vi "adjust_default_pressure.vi"(11 "Set Pressure Cluster":T1={"Control Pressure"=268.93469325770803, "Set Water Mix Pressures"=[nan, nan, nan, 501.0563822038507, 515.6849104636661, 529.5698810290002, 543.7581328797552, 555.1850771044066, 568.1044613714394], "Set Odor Pressures"=[nan, nan, 465.17755108085316, 474.38001525731295]}) -> (3 "new default pressure":dbl[](array[numeric]))   [LabVIEW 2016]
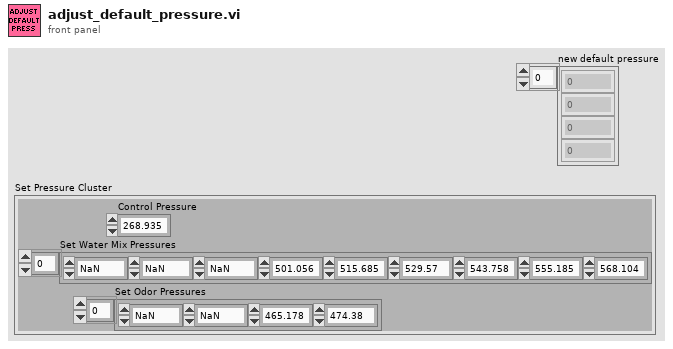
[diagram p1: front panel]
types:
  T1 = cluster{"Control Pressure":dbl, "Set Water Mix Pressures":dbl[], "Set Odor Pressures":dbl[]}
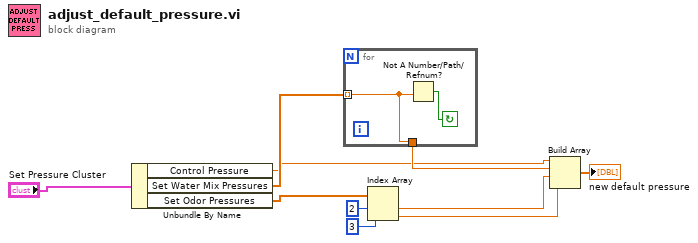
[diagram p0: block diagram]
diagram:
  n1 = Unbundle By Name("Set Pressure Cluster") -> ("Control Pressure"=w2:dbl, "Set Water Mix Pressures"=w4:dbl[], "Set Odor Pressures"=w9:dbl[])
  n2 = for {
    tunnel: w4 -> [w11] mode=indexing
    tunnel: [w11] -> w3
    stop <- w12 continue-if-true
    n3 = Not A Number/Path/Refnum?(number/path/refnum=w11) -> (NaN/Path/Refnum?=w12:bool)
  }
  n4 = Index Array(array=w9, index #1=2 ("index"), index #2=3 ("index")) -> (element #1=w6:dbl, element #2=w5:dbl)
  n5 = Build Array(w2, w3, w6, w5) -> (→"new default pressure":dbl[])
